vi "Switch Warning.vi"(1 "Air Dry Switch":bool, 2 "Main Wash Switch":bool, 3 "Underbody Switch A":bool) -> (0 "Switch Warning":bool)   [LabVIEW 2024]
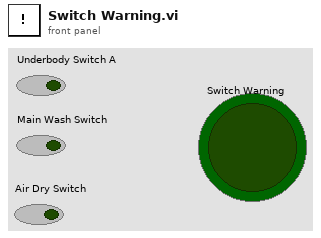
[diagram p1: front panel]
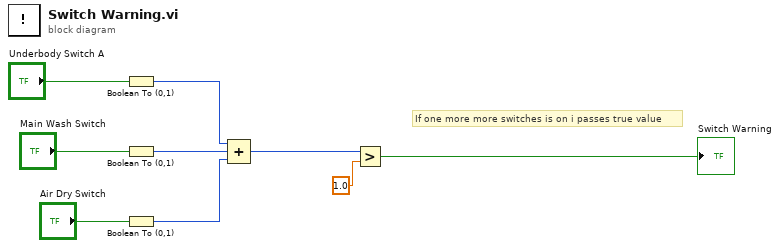
[diagram p0: block diagram]
diagram:
  # "If one more more switches is on i passes true value"
  n1 = Boolean To (0,1)(Boolean="Underbody Switch A") -> (0, 1=w9:i16)
  n2 = Boolean To (0,1)(Boolean="Main Wash Switch") -> (0, 1=w8:i16)
  n3 = Boolean To (0,1)(Boolean="Air Dry Switch") -> (0, 1=w7:i16)
  n4 = Compound Arithmetic op=ADD(w9, w8, w7) -> (w6:i16)
  n5 = Greater?(x=w6, y=1.0) -> (0:→"Switch Warning":bool)
